vi "deglitcher.vi"(1 "Pin":refnum<k21>="SDA0") -> (0 "Result":bool)   [LabVIEW 2010]
uses:
  <vilib>/eio/EIONode/EIONode.xnode
  <vilib>/rvi/eio/nirviEIOImplementation/nirviEIOImplementation.xnode
  <vilib>/rvi/eio/common/nirviEmuClasses.ctl
  <vilib>/rvi/eio/common/nirviEmuTemplateMethod_noerrors.vi
panel:
  in  "State":fxp<+/-,3,3>=-4.0
  # "Read digital input, deglitching by four cycle delay (four invocations)"
  # "Local variable:"
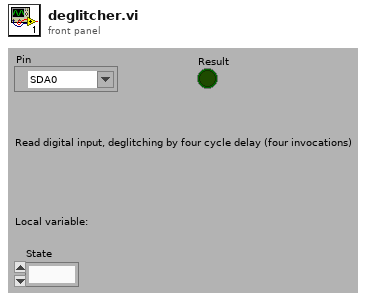
[diagram p1: front panel]
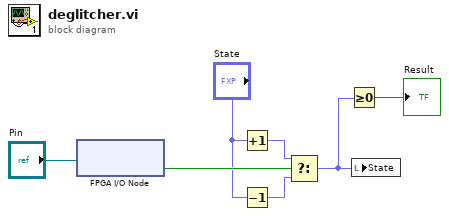
[diagram p0: block diagram]
diagram:
  n1 = xnode "FPGA I/O Node"("FPGA I/O In"="Pin") -> ("I/O Item"=w6:bool)  [unwired: 1 out]
  n2 = Increment(x="State") -> (x+1=w4:fxp<+/-,3,3>)
  n3 = Decrement(x="State") -> (x-1=w5:fxp<+/-,3,3>)
  n4 = Select(t=w4, s=w6, f=w5) -> (s? t:f=w2:fxp<+/-,3,3>)
  n5 = Greater Or Equal To 0?(x=w2) -> (x >= 0?=→"Result":bool)
  n6 = local write "State"(w2) -> ()
